vi "Read Measurement (Spectrum Emission Mask).vi"(0 "VISA resource name":refnum<visa-resource-name>, 11 "error in (no error)":errorcluster) -> (4 "VISA resource name out":refnum<visa-resource-name>, 6 "SEM Measurement":T1 {"Lower_offset6" format="%.3f"; "Lower_offset5" format="%.3f"; "Lower_offset4" format="%.3f"; "Lower_offset3" format="%.3f"; "Lower_offset2" format="%.3f"; "Lower_offset1" format="%.3f"; "Upper_offset6" format="%.3f"; "Upper_offset5" format="%.3f"; "Upper_offset4" format="%.3f"; "Upper_offset3" format="%.3f"; "Upper_offset2" format="%.3f"; "Upper_offset1" format="%.3f"; "Margin_Upper_offset6" format="%.3f"; "Margin_Lower_offset6" format="%.3f"; "Abs_Upper_offset6" format="%.3f"; "Abs_Lower_offset6" format="%.3f"; "Margin_Upper_offset5" format="%.3f"; "Margin_Lower_offset5" format="%.3f"; "Abs_Upper_offset5" format="%.3f"; "Abs_Lower_offset5" format="%.3f"; "Margin_Upper_offset4" format="%.3f"; "Margin_Lower_offset4" format="%.3f"; "Abs_Upper_offset4" format="%.3f"; "Abs_Lower_offset4" format="%.3f"; "Margin_Upper_offset3" format="%.3f"; "Margin_Lower_offset3" format="%.3f"; "Abs_Upper_offset3" format="%.3f"; "Abs_Lower_offset3" format="%.3f"; "Margin_Upper_offset2" format="%.3f"; "Margin_Lower_offset2" format="%.3f"; "Abs_Upper_offset2" format="%.3f"; "Abs_Lower_offset2" format="%.3f"; "Margin_Upper_offset1" format="%.3f"; "Margin_Lower_offset1" format="%.3f"; "Abs_Upper_offset1" format="%.3f"; "Abs_Lower_offset1" format="%.3f"; "Reference" format="%.3f"; "Judgement Result" items=["PASS", "FAIL"]}, 15 "error out":errorcluster)   [LabVIEW 2020, in "Anritsu Signal Analyzer Series.lvlib"]
doc: "Reads Spectrum Emission Mask measurement Data."
uses:
  Anritsu Signal Analyzer Series.lvlib
panel:
  # "dBm"
  # "Upper"
  # "Lower"
  # "Margin(dB)"
  # "Frequency(Hz)"
  # "Offset(dB)"
  # "Peak(dBm)"
  # "Margin(dB)"
  # "Frequency(Hz)"
  # "Offset(dB)"
  # "Peak(dBm)"
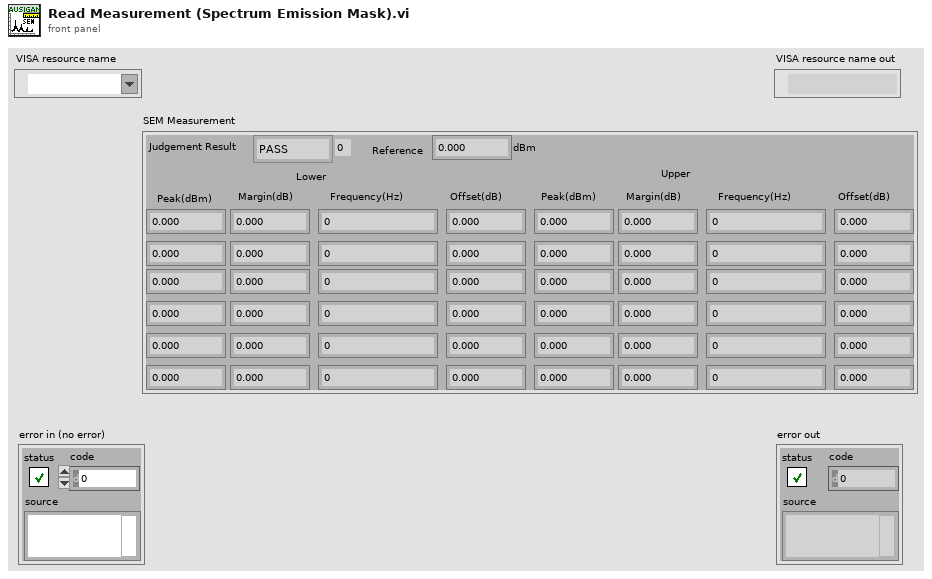
[diagram p1: front panel]
types:
  T1 = cluster{"Judgement Result":dbl, "Reference":dbl, "Abs_Lower_offset1":dbl, "Margin_Lower_offset1":dbl, "Freq_Lower_Offset1":dbl, "Lower_offset1":dbl, "Abs_Upper_offset1":dbl, "Margin_Upper_offset1":dbl, "Freq_Upper_Offset1":dbl, "Upper_offset1":dbl, "Abs_Lower_offset2":dbl, "Margin_Lower_offset2":dbl, "Freq_Lower_Offset2":dbl, "Lower_offset2":dbl, "Abs_Upper_offset2":dbl, "Margin_Upper_offset2":dbl, "Freq_Upper_Offset2":dbl, "Upper_offset2":dbl, "Abs_Lower_offset3":dbl, "Margin_Lower_offset3":dbl, "Freq_Lower_Offset3":dbl, "Lower_offset3":dbl, "Abs_Upper_offset3":dbl, "Margin_Upper_offset3":dbl, "Freq_Upper_Offset3":dbl, "Upper_offset3":dbl, "Abs_Lower_offset4":dbl, "Margin_Lower_offset4":dbl, "Freq_Lower_Offset4":dbl, "Lower_offset4":dbl, "Abs_Upper_offset4":dbl, "Margin_Upper_offset4":dbl, "Freq_Upper_Offset4":dbl, "Upper_offset4":dbl, "Abs_Lower_offset5":dbl, "Margin_Lower_offset5":dbl, "Freq_Lower_Offset5":dbl, "Lower_offset5":dbl, "Abs_Upper_offset5":dbl, "Margin_Upper_offset5":dbl, "Freq_Upper_Offset5":dbl, "Upper_offset5":dbl, "Abs_Lower_offset6":dbl, "Margin_Lower_offset6":dbl, "Freq_Lower_Offset6":dbl, "Lower_offset6":dbl, "Abs_Upper_offset6":dbl, "Margin_Upper_offset6":dbl, "Freq_Upper_Offset6":dbl, "Upper_offset6":dbl}
  T2 = cluster{"[0]":dbl, "[1]":dbl, "[2]":dbl, "[3]":dbl, "[4]":dbl, "[5]":dbl, "[6]":dbl, "[7]":dbl, "[8]":dbl, "[9]":dbl, "[10]":dbl, "[11]":dbl, "[12]":dbl, "[13]":dbl, "[14]":dbl, "[15]":dbl, "[16]":dbl, "[17]":dbl, "[18]":dbl, "[19]":dbl, "[20]":dbl, "[21]":dbl, "[22]":dbl, "[23]":dbl, "[24]":dbl, "[25]":dbl, "[26]":dbl, "[27]":dbl, "[28]":dbl, "[29]":dbl, "[30]":dbl, "[31]":dbl, "[32]":dbl, "[33]":dbl, "[34]":dbl, "[35]":dbl, "[36]":dbl, "[37]":dbl, "[38]":dbl, "[39]":dbl, "[40]":dbl, "[41]":dbl, "[42]":dbl, "[43]":dbl, "[44]":dbl, "[45]":dbl, "[46]":dbl, "[47]":dbl, "[48]":dbl, "[49]":dbl}
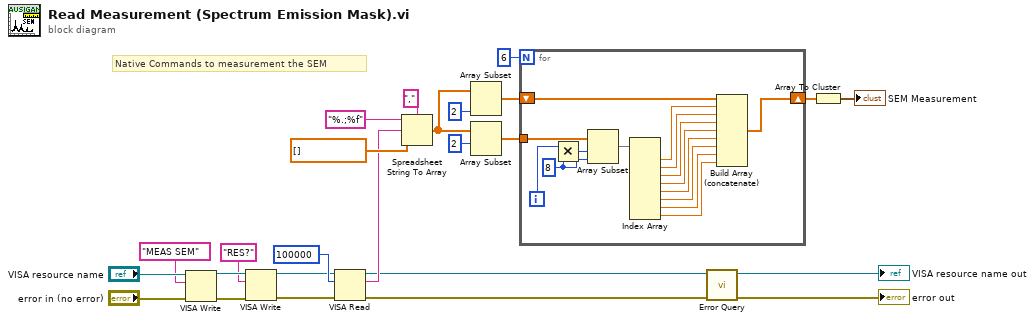
[diagram p0: block diagram]
diagram:
  # "Native Commands to measurement the SEM"
  n1 = VISA Write(VISA resource name="VISA resource name", write buffer="MEAS SEM" ("_CommandSet"), error in (no error)="error in (no error)") -> (VISA resource name out=w8:refnum<visa-resource-name>, error out=w7:errorcluster)  [unwired: 1 out]
  n2 = VISA Write(VISA resource name=w8, write buffer="RES?" ("_Command"), error in (no error)=w7) -> (VISA resource name out=w9:refnum<visa-resource-name>, error out=w10:errorcluster)  [unwired: 1 out]
  n3 = VISA Read(VISA resource name=w9, byte count=u32 100000 ("byte count (0)"), error in (no error)=w10) -> (VISA resource name out=w3:refnum<visa-resource-name>, read buffer=w6:string, error out=w4:errorcluster)  [unwired: 1 out]
  n4 = Spreadsheet String To Array(delimiter (Tab)=",", format string="%.;%f", spreadsheet string=w6, array type (2D Dbl)=dbl[] [] ("Values")) -> (array=w5:dbl[])
  n5 = Array Subset(array=w5, length=2 ("長さ")) -> (w17:dbl[])  [unwired: 1 in]
  n6 = Array Subset(array=w5, index=2 ("長さ")) -> (w19:dbl[])  [unwired: 1 in]
  n7 = for {
    N: 6 -> [_]
    tunnel: w19 -> [w40]
    shift-right: [w28] -> w16
    shift-left: w17 -> [w35]
    i -> [w39]
    w38 = 8 ("長さ")
    n8 = Multiply(x=w39, y=w38) -> (x*y=w37:i32)
    n9 = Array Subset(array=w40, index=w37, length=w38) -> (w36:dbl[])
    n10 = Index Array(array=w36) -> (element #1=w34:dbl, element #2=w33:dbl, element #3=w26:dbl, element #4=w32:dbl, element #5=w31:dbl, element #6=w30:dbl, element #7=w27:dbl, element #8=w29:dbl)  [unwired: 8 in]
    n11 = Build Array (concatenate)(w35, w34, w33, w26, w32, w31, w30, w27, w29) -> (w28:dbl[])
  }
  n12 = call "Error Query.vi"("error in (no error)"=w4, "VISA resource name"=w3) -> ("error out"=→"error out":errorcluster, "VISA resource name out"=→"VISA resource name out":refnum<visa-resource-name>)  [unwired: 6 in, 2 out]
  n13 = Array To Cluster(array=w16) -> (cluster=→"SEM Measurement":T2)
